vi "FEA_Model_Online_Solver.vi"(8 "error in (no error)":errorcluster, 11 "FEA_Model in":refnum<class "FEA_Model.lvclass">) -> (0 "error out":errorcluster, 3 "FEA_Model out":refnum<class "FEA_Model.lvclass">)   [LabVIEW 2021, in "FEA_Model.lvclass"]
uses:
  FEA_Model.lvclass
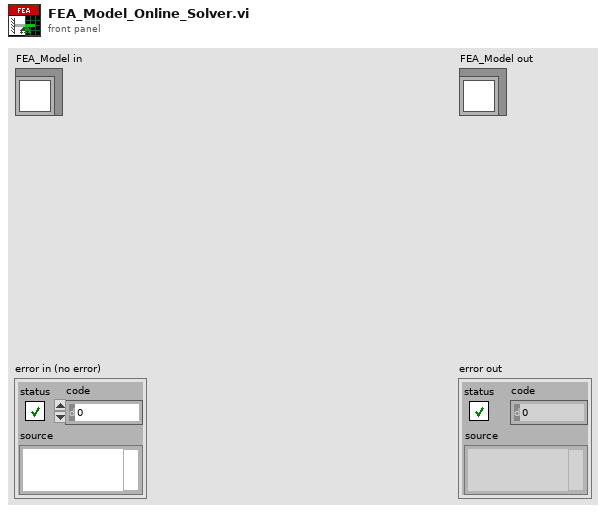
[diagram p1: front panel]
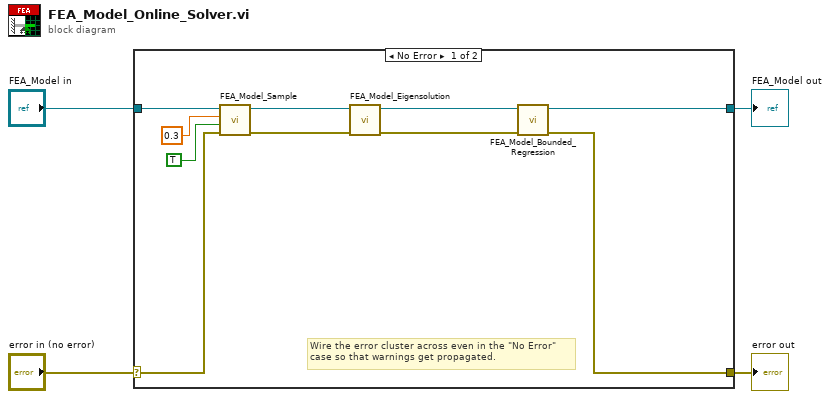
[diagram p0: block diagram]
diagram:
  n1 = case shown="No Error" "error in (no error)" {
    selector: "error in (no error)" -> [w6 w16]
    tunnel: [w5 w16] -> w3
    tunnel: [w9 w15] -> w1
    tunnel: "FEA_Model in" -> [w14 w15]
    frame No Error {
      # "Wire the error cluster across even in the \"No Error\"\ncase so that warnings get propagated."
      n2 = call-dynamic "FEA_Model_Sample.vi"("error in (no error)"=w6, "include extremes"=TRUE, "standard_deviation"=0.3, "FEA_Model in"=w14) -> ("error out"=w8:errorcluster, "FEA_Model out"=w11:refnum<class "FEA_Model.lvclass">)  [unwired: 6 in]
      n3 = call-dynamic "FEA_Model_Eigensolution.vi"("error in (no error)"=w8, "FEA_Model in"=w11) -> ("error out"=w7:errorcluster, "FEA_Model out"=w10:refnum<class "FEA_Model.lvclass">)  [unwired: 8 in]
      n4 = call-dynamic "FEA_Model_Bounded_Regression.vi"("error in (no error)"=w7, "FEA_Model in"=w10) -> ("error out"=w5:errorcluster, "FEA_Model out"=w9:refnum<class "FEA_Model.lvclass">)  [unwired: 8 in]
    }
    frame Error {
    }
  }
  "error out" <- w3
  "FEA_Model out" <- w1
